vi "DAQ 1SDI v6.1_whale_a.vi"() -> ()   [LabVIEW 2013]
uses:
  Strict Type Defs/type_meas_enum.ctl
  <instrlib>/niScope/Controls/niScope vertical coupling.ctl
panel:
  out "covariance HD 2 & 6":waveform(dbl)(graph)
  out "covariance HD 2 & 4":waveform(dbl)(graph)
  out "covariance HD 2 & 5":waveform(dbl)(graph)
  in  "stop":bool
  out "Loop count":i32=4690
  in  "Monitors":enum32{"Monitors On", "Monitors Off"}(tab)
  out "covariance HD 1 & 2":dbl(graph)=0.19831028169384832
  out "Conditional variance HD 1|2":dbl(graph)=1.0142124161365378
  out "Conditional variance HD 1|3":dbl(graph)=0.6065160666682574
  out "Conditional variance HD 2|3":dbl(graph)=0.5661489724627885
  out "covariance HD 1 & 3":dbl(graph)=-0.6559385878875881
  out "covariance HD 2 & 3":dbl(graph)=-0.6106758756892631
  in  "Settings":enum32{"Settings and Record", "Under the hood"}(tab)=enum."Under the hood"
  in  "Knob":u32(knob)=43 scale=0.0..250.0
  in  "Number of monitor samples":i32=10000 format="%.0p"
  in  "File location":path=path "C:/ni-rt/LabVIEW Data/July1/35dB109"
  in  "Type of measurement":T1=enum."electronic"
  in  "File root name":string="Real"
  in  "Number of samples save":i32=2000000 format="%.0p"
  in  "reset sn":bool
  in  "Shot noise start":bool
  in  "Additional text":string="OPA 1 optical power set to 15mV on HD A.\nOPA 2 optical power set to 15mV on HD B.\nLocal oscillator is set to 5V on HD.\nParametric gain set to 15 for OPA 1.\nParametric gain set to 15 for OPA 2.\nVertical range set to 0.5V for both channels.\nSample rate set to 14MS/s.\nMax input freq set to7MHz.\nVisibility between OPA 1 & OPA 2 = 99.6\nVisibility between OPA 1 & L.O.B = 98.9\nVisibility between OPA 1 & L.O. A = 98.9\nBoth squeezers expected to produce -7dB/11dB.\nLoss on EPR B =55.33% (3.5dB) \n"
  in  "Record":bool
  in  "Number of Files":i32=2
  out "File count":i32=1
  in  "Run":string="9"
  out "Cluster":T2={"Actual samples acquired ch 1"=120000, "Actual samples acquired ch 0"=120000, "Actual samples acquired ch 2"=120000}
  in  "Channel Parms":T4={"Input impedance (Ohms)"=2, "Maximum input frequency (Hz)"=7.0, "vertical coupling"=1, "Probe attenuation"=1.0, "Vertical range (V)"=1.0, "Vertical offset"=0.0, "channel enabled"=TRUE} {"Input impedance (Ohms)" items=["1 mega ohm"=0, "50 ohms"=2]; "Maximum input frequency (Hz)" format="%#_6p"; "vertical coupling" items=["AC", "DC", "Ground"]}
  in  "IIR filter specifications":T5={"Topology"=enum."Butterworth", "Type"=enum."Bandpass", "Order"=6, "Lower Fc"=2900000.0, "Upper Fc"=3100000.0, "PB Ripple"=1.0, "SB Attenuation"=60.0} {"PB Ripple" format="%0.2f"; "SB Attenuation" format="%0.2f"; "Lower Fc" format="%0.2p"; "Upper Fc" format="%0.2p"}
  out "error out":errorcluster caption="error out final"
  in  "max time (s)":dbl=10.0 caption="Time to run (s)"
  in  "Reference position":dbl(slide)=50.0 scale=0.0..100.0
  in  "Minimum sample rate (S/s)":dbl=14000000.0 format="%#_6p"
  out "Video bandwidth (Hz)":dbl=7.0
  in  "DAQ Cards":T6={"DAQ Card 1"="Dev2", "DAQ Card 2"="Dev3"}
  # "Variance won't be displayed until shot noise is taken"
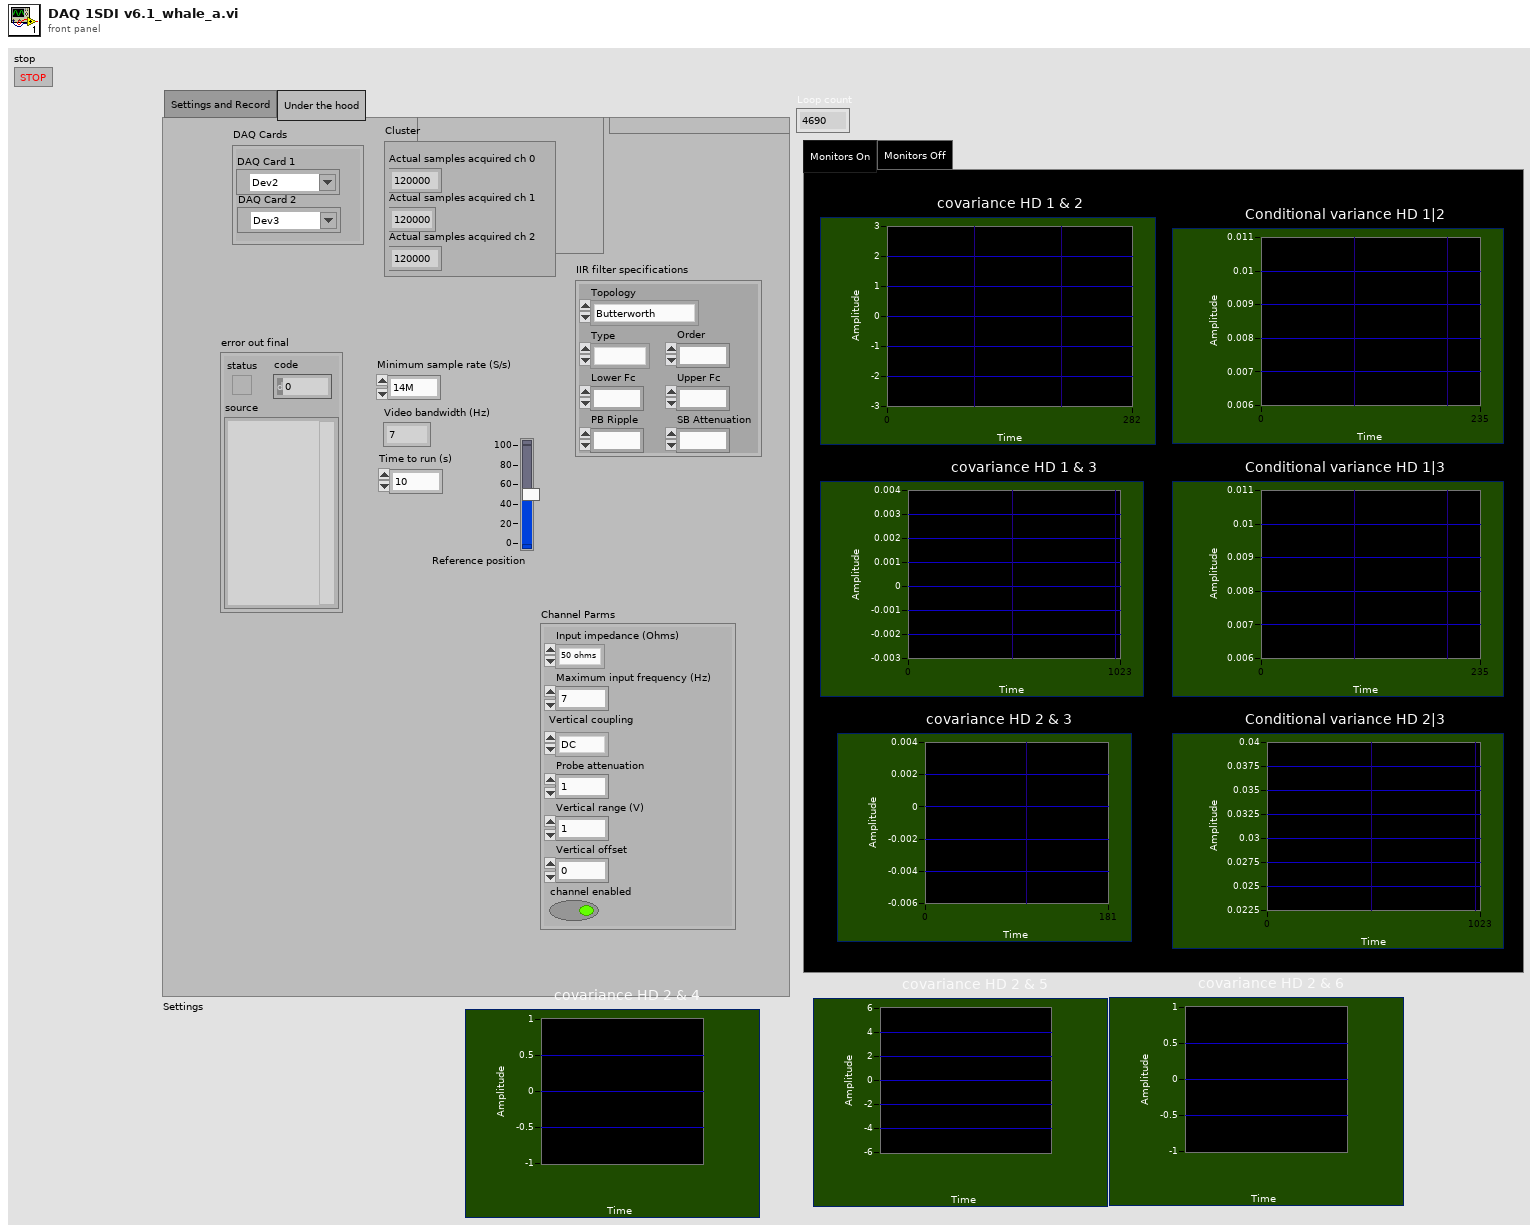
[diagram p1: front panel]
types:
  T1 = typedef "type_meas_enum.ctl" = enum16{"shot", "x", "p", "electronic"}
  T2 = cluster{"Actual samples acquired ch 1":i32, "Actual samples acquired ch 0":i32, "Actual samples acquired ch 2":i32}
  T3 = typedef "niScope vertical coupling.ctl" = i32
  T4 = cluster{"Input impedance (Ohms)":u32, "Maximum input frequency (Hz)":dbl, "vertical coupling":T3, "Probe attenuation":dbl, "Vertical range (V)":dbl, "Vertical offset":dbl, "channel enabled":bool}
  T5 = cluster{"Topology":enum16{"Off", "Butterworth", "Chebyshev", "Inverse Chebyshev", "Elliptic", "Bessel"}, "Type":enum16{"Lowpass", "Highpass", "Bandpass", "Bandstop"}, "Order":i32, "Lower Fc":dbl, "Upper Fc":dbl, "PB Ripple":dbl, "SB Attenuation":dbl}
  T6 = cluster{"DAQ Card 1":refnum<k15>, "DAQ Card 2":refnum<k15>}
  T7 = cluster{"instrument handle":refnum<k15>, "instrument handle":refnum<k15>}
  T8 = cluster{"instrument handle out 0":refnum<k15>, "instrument handle out 1":refnum<k15>}
  T9 = cluster{"actualSamples":i32, "actualSamples":i32, "actualSamples":i32}
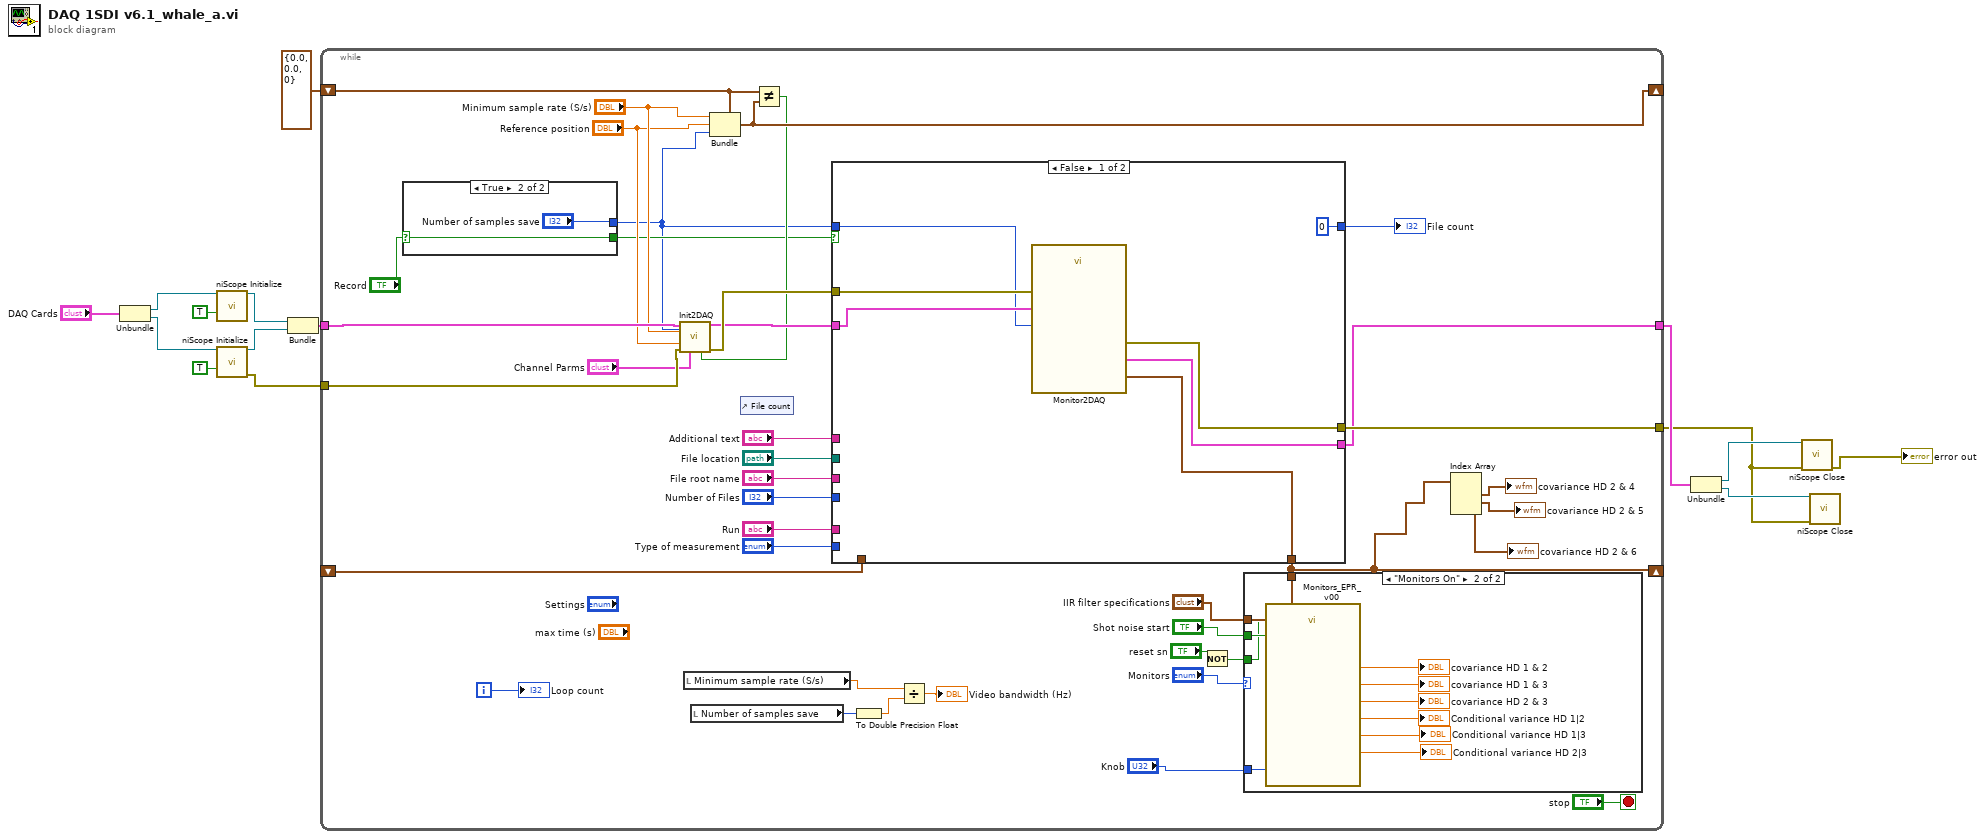
[diagram p0: block diagram]
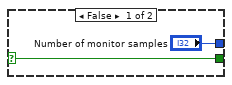
[diagram p2: hidden frame]
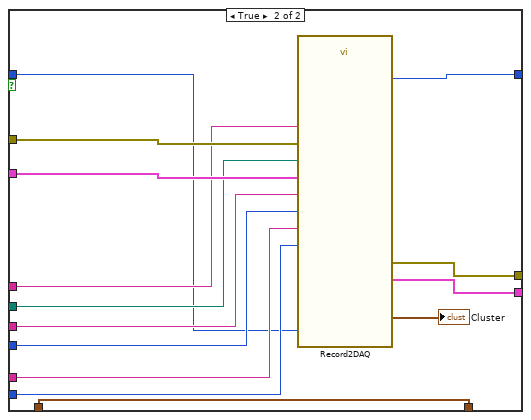
[diagram p4: hidden frame]
diagram:
  n1 = Unbundle("DAQ Cards") -> ("DAQ Card 1"=w7:refnum<k15>, "DAQ Card 2"=w6:refnum<k15>)
  n2 = call <instrlib>:"niScope Initialize.vi"("resource name"=w7, "reset device"=TRUE) -> ("instrument handle"=w4:refnum<k15>)  [unwired: 12 in, 1 out]
  n3 = call <instrlib>:"niScope Initialize.vi"("resource name"=w6, "reset device"=TRUE) -> ("instrument handle"=w3:refnum<k15>, "error out"=w5:errorcluster)  [unwired: 12 in]
  n4 = Bundle("instrument handle"=w4, "instrument handle"=w3) -> (w2:T7)  [unwired: 1 in]
  n5 = while {
    tunnel: [w48] -> w11
    tunnel: w5 -> [w34]
    shift-right: [w29] -> _
    shift-left: cluster{dbl, dbl, i32} {0.0, 0.0, 0} -> [w30]
    shift-right: [w20] -> _
    shift-left: _ -> [w24]
    tunnel: w2 -> [w35]
    tunnel: [w37] -> w15
    i -> [w50]
    stop <- "stop" stop-if-true
    n6 = case shown="True" "Record" {
      selector: "Record" -> [w56 w58]
      tunnel: ["Number of monitor samples" "Number of samples save"] -> w21
      tunnel: [w56 w58] -> w25
      frame False {
      }
      frame True {
      }
    }
    n7 = local read "Minimum sample rate (S/s)"() -> (w38:dbl)
    n8 = local read "Number of samples save"() -> (w40:i32)
    n9 = Bundle(cluster=w30, "Minimum sample rate (S/s)", "Reference position", w21) -> (w29:cluster{dbl, dbl, i32})
    n10 = control-ref of="File count"() -> ()  [unwired: 1 out]
    n11 = Not Equal?(x=w30, y=w29) -> (x != y?=w28:bool)
    n12 = call "Init2DAQ.vi"("resource names"=w35, "min record length"=w21, "min sample rate"="Minimum sample rate (S/s)", "reference position"="Reference position", "error in"=w34, "channel parms"="Channel Parms", "Ch param"=w28) -> ("instrument out"=w36:T8, "error out"=w54:errorcluster)  [unwired: 7 in]
    n13 = case shown="False" w25 {
      tunnel: w36 -> [w75 w90]
      tunnel: w54 -> [w76 w89]
      tunnel: [w74 w88] -> w48
      tunnel: "Additional text" -> [_ w87]
      tunnel: "File location" -> [_ w86]
      tunnel: "File root name" -> [_ w85]
      tunnel: "Number of Files" -> [_ w84]
      tunnel: "Run" -> [_ w83]
      tunnel: "Type of measurement" -> [_ w82]
      tunnel: [w73 w79] -> w20
      tunnel: [w72 w80] -> w37
      tunnel: w24 -> [_ w79]
      tunnel: w21 -> [w71 w78]
      tunnel: [0 ("File count") w77] -> w16
      frame False {
        n14 = call "Monitor2DAQ.vi"("instrument in"=w75, "error in"=w76, "numSamples"=w71) -> ("instrument out"=w72:T8, "wfm"=w73:waveform(dbl)[], "error out"=w74:errorcluster)  [unwired: 10 in]
      }
      frame True {
        n15 = call "Record2DAQ.vi"("instrument in"=w90, "Additional text"=w87, "numSamples"=w78, "File location"=w86, "Type of\nmeasurement"=w82, "Name root"=w85, "error in"=w89, "Run"=w83, "number of files"=w84) -> ("output cluster"=→"Cluster":T9, "instrument out"=w80:T8, "File count"=w77:i32, "error out"=w88:errorcluster)  [unwired: 2 in, 1 out]
      }
    }
    "File count" <- w16
    n16 = To Double Precision Float(number=w40) -> (double precision float=w39:dbl)
    n17 = Divide(x=w38, y=w39) -> (x/y=→"Video bandwidth (Hz)":dbl)
    n18 = Not(x="reset sn") -> (.not. x?=w33:bool)
    n19 = case shown="\"Monitors On\"" "Monitors" {
      tunnel: "Shot noise start" -> [_ w69]
      tunnel: "IIR filter specifications" -> [_ w68]
      tunnel: w33 -> [_ w67]
      tunnel: w20 -> [_ w66]
      tunnel: "Knob" -> [_ w59]
      frame "Monitors Off" {
      }
      frame "Monitors On" {
        n20 = call "Monitors_EPR_v00.vi"("IIR filter specifications"=w68, "Wait(mSec)"=w59, "reset SN"=w67, "Shot noise start"=w69, "wfm"=w66) -> ("covariance B01"=→"covariance HD 1 & 2":dbl, "covariance B0A"=→"covariance HD 1 & 3":dbl, "covariance B1A"=→"covariance HD 2 & 3":dbl, "conditional variance B0|1"=→"Conditional variance HD 1|2":dbl, "conditional variance B1|A"=→"Conditional variance HD 2|3":dbl, "conditional variance B0|A"=→"Conditional variance HD 1|3":dbl)  [unwired: 5 in]
      }
    }
    n21 = Index Array(array=w20) -> (element #1=→"covariance HD 2 & 4":waveform(dbl), element #2=→"covariance HD 2 & 5":waveform(dbl), element #3=→"covariance HD 2 & 6":waveform(dbl))  [unwired: 3 in]
    "Loop count" <- w50
  }
  n22 = Unbundle(w15) -> ("instrument handle out 0"=w14:refnum<k15>, "instrument handle out 1"=w13:refnum<k15>)
  n23 = call <instrlib>:"niScope Close.vi"("instrument handle"=w14, "error in"=w11) -> ("error out"=→"error out":errorcluster)  [unwired: 13 in]
  n24 = call <instrlib>:"niScope Close.vi"("instrument handle"=w13, "error in"=w11) -> ()  [unwired: 13 in, 1 out]
